vi "Method.vi"(4 "Input B":refnum<class "Abs_Numeric.lvclass">, 5 "Input A":T1) -> (1 "Result":T1)   [LabVIEW 2021, in "Add_I64.lvclass"]
uses:
  Add_I64.lvclass
  Abs_Type.ctl
  Abs_Types/I64 Integer/Abs_I64 Integer.lvclass
  Abs_Types/Numeric/Abs_Numeric.lvclass
  C:/Users/Tim/Documents/LabVIEW/2021/Data Classes/Source/Functions/Support/Two Terminal/I64/AbsFunc_Two Term_I64.lvclass
  C:/Users/Tim/Documents/LabVIEW/2021/Data Classes/Source/Abs_Types/I64 Integer/Abs_I64 Integer.lvclass
  Support/Two Terminal/I64/AbsFunc_Two Term_I64.lvclass/AbsFunc_Two Term_I64.ctl
  Support/Two Terminal/I64/Properties/Write Numeric A.vi
  Support/Two Terminal/I64/Properties/Write Numeric B.vi
  Add_I64.lvclass/Add_I64.ctl
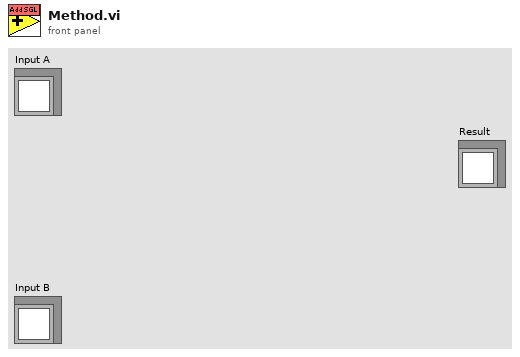
[diagram p1: front panel]
types:
  T1 = typedef "Add_I64.lvclass/Abs_Type.ctl" = refnum<class "Abs_I64 Integer.lvclass">
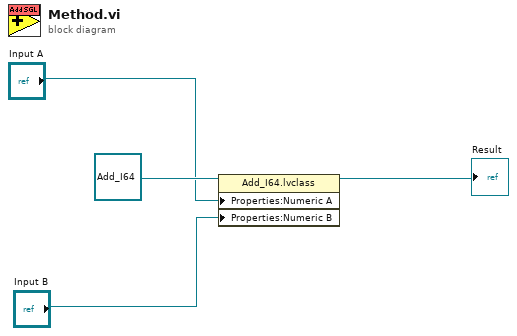
[diagram p0: block diagram]
diagram:
  n1 = property class="Add_I64.lvclass"(reference=refnum<class "Add_I64.lvclass"> refnum ("Functions.lvlib:Numeric.lvlib:Add_SGL.lvclass"), "Properties:Numeric A"="Input A", "Properties:Numeric B"="Input B") -> (reference out=→"Result":refnum<class "Add_I64.lvclass">)  [unwired: 1 in, 1 out]
